vi "Window_pulses.vi"(10 "beta":dbl, 11 "Pulses":waveform(dbl)[](array[waveform])) -> (3 "Array":waveform(dbl)[](array[waveform]))   [LabVIEW 2015]
uses:
  <vilib>/Analysis/4window.llb/Kaiser-Bessel Window (DBL).vi
  <vilib>/Analysis/NI_AALPro.lvlib
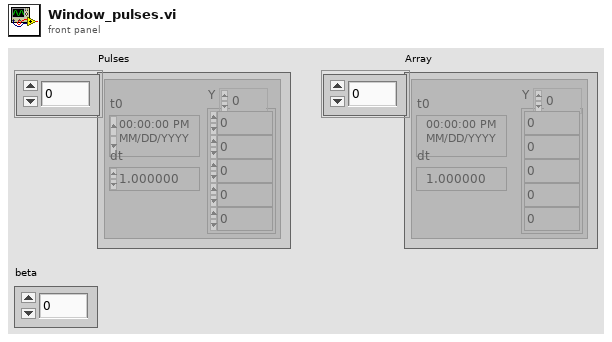
[diagram p1: front panel]
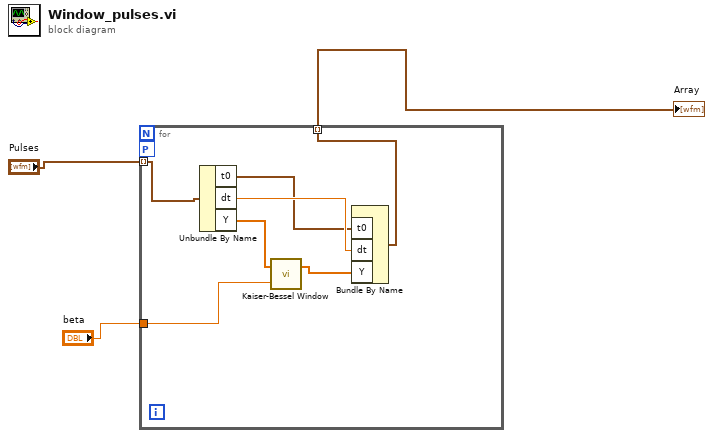
[diagram p0: block diagram]
diagram:
  n1 = for {
    tunnel: "Pulses" -> [w10] mode=indexing
    tunnel: [w6] -> w2 mode=indexing
    workers-P: _ -> [_]
    tunnel: "beta" -> [w4]
    n2 = Unbundle By Name(w10) -> ("t0"=w5:timestamp, "dt"=w7:dbl, "Y"=w9:dbl[])
    n3 = call-poly <vilib>:"Kaiser-Bessel Window.vi"("beta"=w4, "X"=w9) -> ("Windowed X"=w8:dbl[])  [unwired: 1 out]
    n4 = Bundle By Name("t0"=w5, "dt"=w7, "Y"=w8) -> (w6:waveform(dbl))  [unwired: 1 in]
  }
  "Array" <- w2
